vi "subArraycheck.vi"(10 "type":T1(ring)=enum."QSFP28", 11 "source":string[](array[string])) -> (0 "is in?":bool, 3 "diff element":string[](array[string]))   [LabVIEW 2011]
uses:
  <userlib>/_OpenG.lib/array/array.llb/Filter 1D Array (String)__ogtk.vi
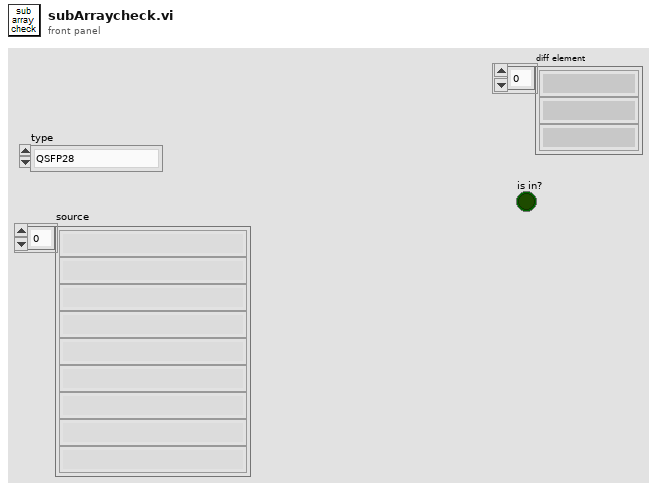
[diagram p1: front panel]
types:
  T1 = enum16{"MINI SAS HD 4X", "MINI SAS 4X", "SFP28", "QSFP28", "SFP+", "SLIM"}
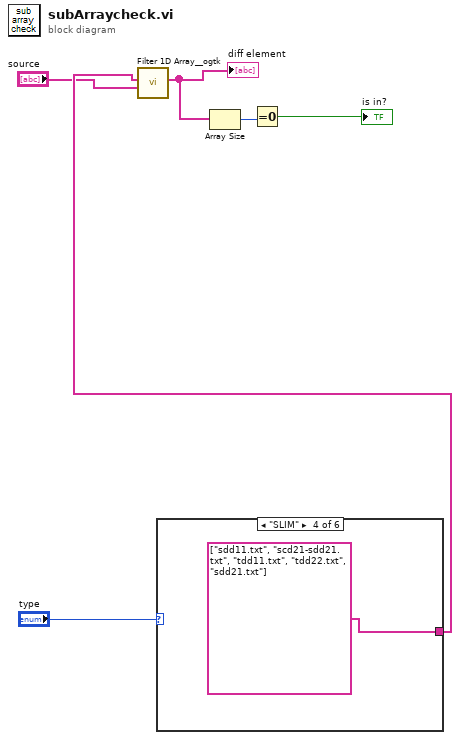
[diagram p0: block diagram]
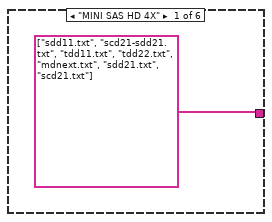
[diagram p2: hidden frame]
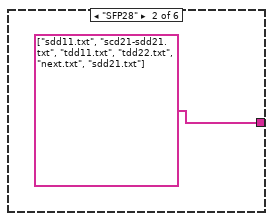
[diagram p3: hidden frame]
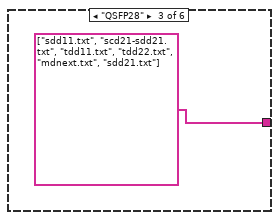
[diagram p4: hidden frame]
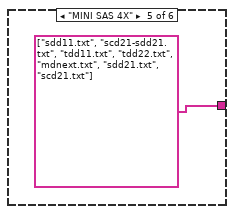
[diagram p5: hidden frame]
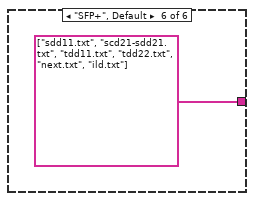
[diagram p6: hidden frame]
diagram:
  n1 = case shown="\"SLIM\"" "type" {
    tunnel: [string[] ["sdd11.txt", "scd21-sdd21.txt", "tdd11.txt", "tdd22.txt", "mdnext.txt", "sdd21.txt", "scd21.txt"] ("target") string[] ["sdd11.txt", "scd21-sdd21.txt", "tdd11.txt", "tdd22.txt", "next.txt", "sdd21.txt"] ("target") string[] ["sdd11.txt", "scd21-sdd21.txt", "tdd11.txt", "tdd22.txt", "mdnext.txt", "sdd21.txt"] ("target") string[] ["sdd11.txt", "scd21-sdd21.txt", "tdd11.txt", "tdd22.txt", "sdd21.txt"] ("target") string[] ["sdd11.txt", "scd21-sdd21.txt", "tdd11.txt", "tdd22.txt", "mdnext.txt", "sdd21.txt", "scd21.txt"] ("target") string[] ["sdd11.txt", "scd21-sdd21.txt", "tdd11.txt", "tdd22.txt", "next.txt", "ild.txt"] ("target")] -> w5
    frame "MINI SAS HD 4X" {
    }
    frame "SFP28" {
    }
    frame "QSFP28" {
    }
    frame "SLIM" {
    }
    frame "MINI SAS 4X" {
    }
    frame "SFP+", Default {
    }
  }
  n2 = call-poly <userlib>:"Filter 1D Array__ogtk.vi"("items to filter"="source", "array"=w5) -> ("filtered array"=w3:string[])  [unwired: 4 in, 1 out]
  "diff element" <- w3
  n3 = Array Size(array=w3) -> (size(s)=w2:i32)
  n4 = Equal To 0?(x=w2) -> (x = 0?=→"is in?":bool)
